vi "Run.vi"(7 "Team Index":i32, 8 "Column":i32, 9 "Row":i32, 10 "View":i32[](array[numeric]) caption="View (Team Index, -1: empty)", 11 "Voyager In":refnum<class "Voyager.lvclass">) -> (0 "Replicated":refnum<class "Square.lvclass">, 1 "Direction":T1, 2 "Action":T2, 3 "Square Out":refnum<class "Square.lvclass">)   [LabVIEW 2015, in "Voyager.lvclass"]
uses:
  Voyager.lvclass
  Square/Square.lvclass
  Type Defs/Action Enum.ctl
  Type Defs/Direction Enum.ctl
  Voyager.lvclass/Voyager.ctl
  SubVIs/Read-Only Globals.vi
  SubVIs/Globals (private).vi
  Common/Common.lvlib
  Type Defs/SB Type Defs.lvlib
panel:
  # "NW\nN\nNE\nE\nSE\nS\nSW\nW"
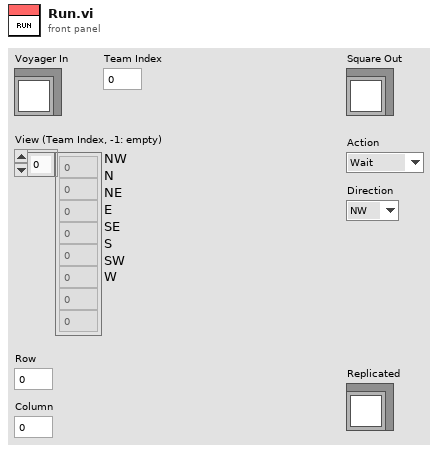
[diagram p1: front panel]
types:
  T1 = typedef "SB Type Defs.lvlib/Direction Enum.ctl" = enum16{"NW", "N", "NE", "E", "SE", "S", "SW", "W"}
  T2 = typedef "SB Type Defs.lvlib/Action Enum.ctl" = enum16{"Wait", "Move", "Attack", "Replicate"}
  T3 = typedef "Common.lvlib/Map DVR.ctl" = refnum<data-value>
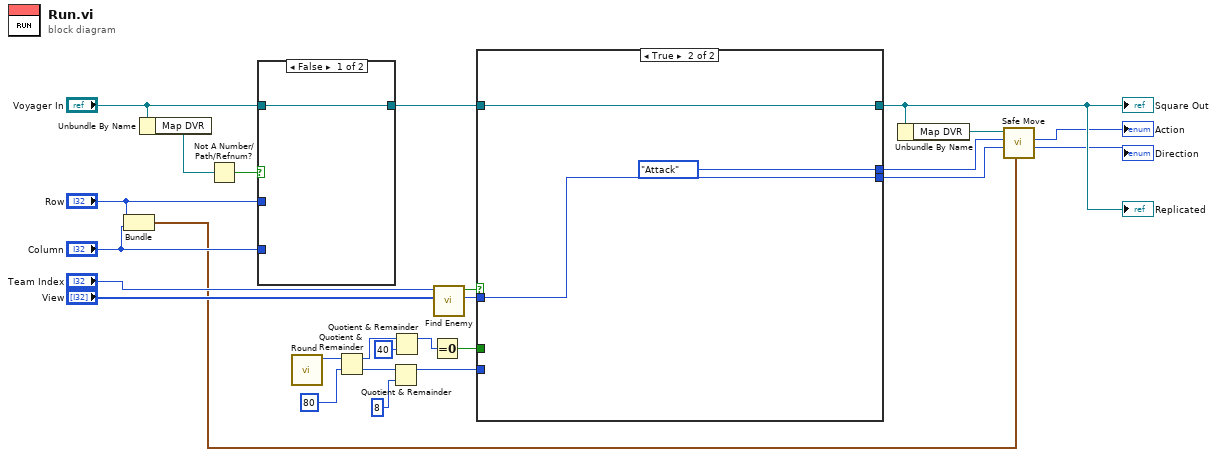
[diagram p0: block diagram]
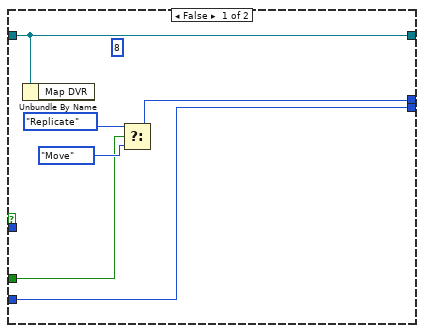
[diagram p2: hidden frame]
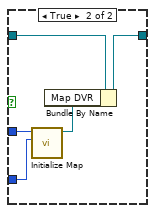
[diagram p3: hidden frame]
diagram:
  n1 = Bundle("Row"="Row", "Column"="Column") -> (w5:cluster{"Row":i32, "Column":i32})  [unwired: 1 in]
  n2 = Unbundle By Name("Voyager In") -> ("Map DVR"=w26:T3)
  n3 = Not A Number/Path/Refnum?(number/path/refnum=w26) -> (NaN/Path/Refnum?=w25:bool)
  n4 = case shown="False" w25 {
    tunnel: "Column" -> [_ w32]
    tunnel: "Row" -> [_ w31]
    tunnel: "Voyager In" -> [w27 w30]
    tunnel: [w27 w28] -> w23
    frame False {
    }
    frame True {
      n5 = call "Initialize Map.vi"("Column"=w32, "Row"=w31) -> ("Map DVR"=w29:T3)  [unwired: 9 in]
      n6 = Bundle By Name(cluster=w30, "Map DVR"=w29) -> (w28:refnum<class "Voyager.lvclass">)
    }
  }
  n7 = call "Round.vi"() -> ("Round"=w21:i32)  [unwired: 11 in]
  n8 = Quotient & Remainder(x=w21, y=80) -> (x-y*floor(x/y)=w11:i32, floor(x/y)=w14:i32)
  n9 = Quotient & Remainder(x=w14, y=8) -> (x-y*floor(x/y)=w12:i32)  [unwired: 1 out]
  n10 = Quotient & Remainder(x=w11, y=40) -> (x-y*floor(x/y)=w9:i32)  [unwired: 1 out]
  n11 = Equal To 0?(x=w9) -> (x = 0?=w8:bool)
  n12 = call "Find Enemy.vi"("View"="View", "Team Index"="Team Index") -> ("Direction"=w17:T1, "Found Enemy?"=w18:bool)  [unwired: 7 in, 1 out]
  n13 = case shown="True" w18 {
    tunnel: [w34 Action_Enum."Attack" ("Action")] -> w4
    tunnel: [w33 w41] -> w3
    tunnel: w23 -> [w38 w39]
    tunnel: w17 -> [_ w41]
    tunnel: [w38 w39] -> w7
    tunnel: w12 -> [w33 _]
    tunnel: w8 -> [w35 _]
    frame False {
      (unwired) 8
      n14 = Unbundle By Name(w38) -> ()  [unwired: 1 out]
      n15 = Select(t=Action_Enum."Replicate" ("Desired Action"), s=w35, f=Action_Enum."Move" ("Desired Action")) -> (s? t:f=w34:T2)
    }
    frame True {
    }
  }
  "Square Out" <- w7
  "Replicated" <- w7
  n16 = Unbundle By Name(w7) -> ("Map DVR"=w6:T3)
  n17 = call "Safe Move.vi"("Position in"=w5, "Direction in"=w3, "Desired Action"=w4, "Map DVR"=w6) -> ("Direction"=→"Direction":T1, "Action"=→"Action":T2)  [unwired: 4 in, 2 out]
